vi "Config_Report.vi"(0 "Previous Pass/Fail":bool=TRUE, 5 "Previous Report Text":string, 7 "Found?":bool, 9 "Key":string, 11 "Section":string) -> (4 "Pass/Fail":bool, 6 "Report Text":string)   [LabVIEW 2023]
doc: "This VI builds the Pass/Fail and report text for parsing config files."
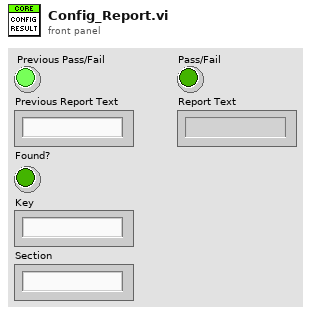
[diagram p1: front panel]
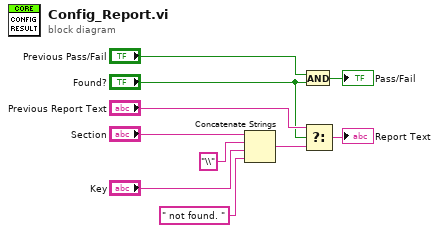
[diagram p0: block diagram]
diagram:
  n1 = Concatenate Strings("Section", "\\" ("string"), "Key", " not found. " ("string")) -> (w8:string)
  n2 = And(x="Previous Pass/Fail", y="Found?") -> (x .and. y?=→"Pass/Fail":bool)
  n3 = Select(t="Previous Report Text", s="Found?", f=w8) -> (s? t:f=→"Report Text":string)
